vi "UMLEditor_GetStereoTypeTemplate.vi"(7 "SubClass":bool, 9 "Connector Pane Pattern":T1=2 items=["4x4x4", "5x6x5", "6x8x6"], 10 "String in":string, 11 "FolderPathOut":path) -> (2 "FoundTemplate":bool, 3 "TemplateToUse":string)   [LabVIEW 2016]
uses:
  <resource>/Framework/Providers/Open_GDS/ClassProviders/Common/ScriptingFunctions/Scripting_ConnectorPanePatternType.ctl
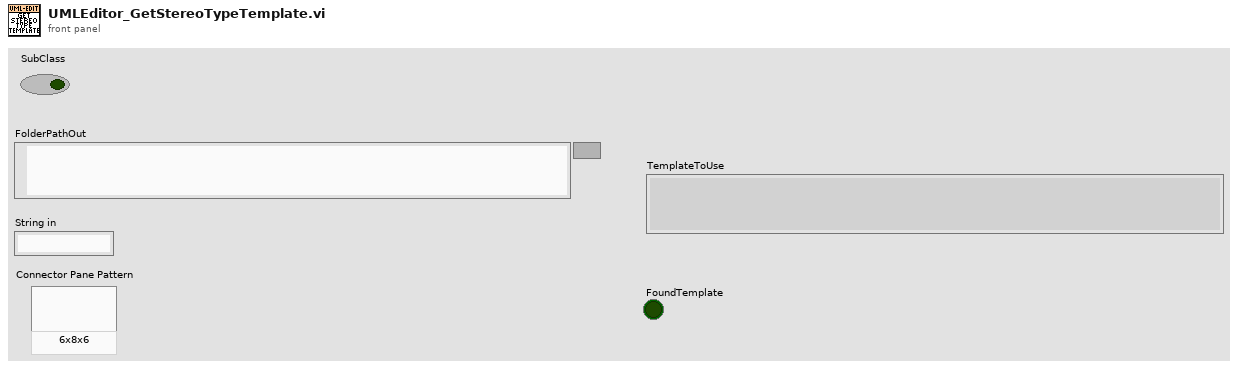
[diagram p1: front panel]
types:
  T1 = typedef "Scripting_ConnectorPanePatternType.ctl" = u16
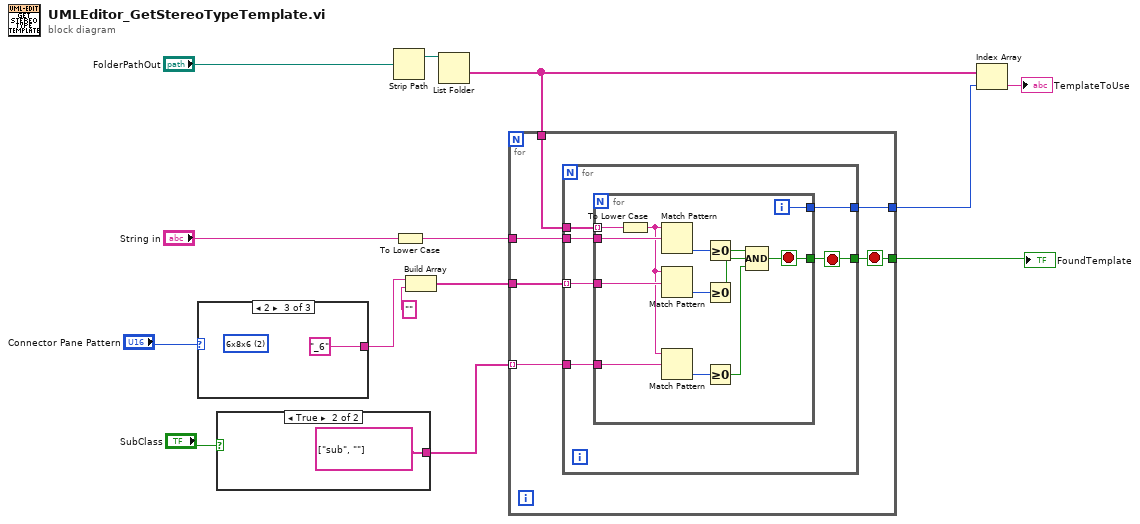
[diagram p0: block diagram]
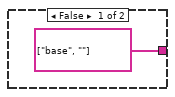
[diagram p2: hidden frame]
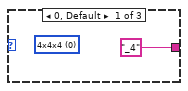
[diagram p3: hidden frame]
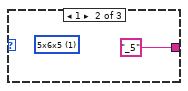
[diagram p4: hidden frame]
diagram:
  n1 = case shown="2" "Connector Pane Pattern" {
    tunnel: ["_4" "_5" "_6"] -> w5
    frame 0, Default {
      (unwired) T1 0 items=["4x4x4", "5x6x5", "6x8x6"] ("Connector Pane Pattern")
    }
    frame 1 {
      (unwired) T1 1 items=["4x4x4", "5x6x5", "6x8x6"] ("Connector Pane Pattern")
    }
    frame 2 {
      (unwired) T1 2 items=["4x4x4", "5x6x5", "6x8x6"] ("Connector Pane Pattern")
    }
  }
  n2 = case shown="True" "SubClass" {
    tunnel: [string[] ["base", ""] string[] ["sub", ""]] -> w1
    frame False {
    }
    frame True {
    }
  }
  n3 = Strip Path(path="FolderPathOut") -> (stripped path=w13:path)  [unwired: 1 out]
  n4 = To Lower Case(string="String in") -> (all lower case string=w11:string)
  n5 = Build Array(w5, "" ("element")) -> (w3:string[])
  n6 = List Folder(path=w13) -> (folder names=w12:string[])  [unwired: 1 in, 5 out]
  n7 = for {
    tunnel: w12 -> [w25]
    tunnel: w11 -> [w24]
    tunnel: [w23] -> w7
    tunnel: [w20] -> w6
    tunnel: w3 -> [w22]
    tunnel: w1 -> [w21] mode=indexing
    stop <- w20 stop-if-true
    n8 = for {
      tunnel: w25 -> [w31]
      tunnel: w24 -> [w30]
      tunnel: [w29] -> w23
      tunnel: [w28] -> w20
      tunnel: w22 -> [w27] mode=indexing
      tunnel: w21 -> [w26]
      stop <- w28 stop-if-true
      n9 = for {
        tunnel: w31 -> [w44] mode=indexing
        tunnel: w30 -> [w43]
        tunnel: [w41] -> w29
        tunnel: [w37] -> w28
        tunnel: w27 -> [w39]
        tunnel: w26 -> [w33]
        i -> [w41]
        stop <- w37 stop-if-true
        n10 = To Lower Case(string=w44) -> (all lower case string=w34:string)
        n11 = Match Pattern(string=w34, regular expression=w43) -> (offset past match=w42:i32)  [unwired: 4 out]
        n12 = Match Pattern(string=w34, regular expression=w39) -> (offset past match=w38:i32)  [unwired: 4 out]
        n13 = Match Pattern(string=w34, regular expression=w33) -> (offset past match=w35:i32)  [unwired: 4 out]
        n14 = Greater Or Equal To 0?(x=w42) -> (x >= 0?=w40:bool)
        n15 = Greater Or Equal To 0?(x=w38) -> (x >= 0?=w36:bool)
        n16 = Greater Or Equal To 0?(x=w35) -> (x >= 0?=w32:bool)
        n17 = Compound Arithmetic op=AND(w40, w36, w32) -> (w37:bool)
      }
    }
  }
  "FoundTemplate" <- w6
  n18 = Index Array(array=w12, index=w7) -> (element=→"TemplateToUse":string)
